vi "Pre Launch Init.vi"(11 "Vision Receiver in":refnum<class "Vision Receiver.lvclass">) -> (0 "error out":errorcluster, 3 "Vision Receiver out":refnum<class "Vision Receiver.lvclass">)   [LabVIEW 2022 SP3, in "Vision.lvlib" / "Vision Receiver.lvlib" / "Vision Receiver.lvclass"]
doc: "(<B>Filename</B>: Actor Framework.lvlib:Actor.lvclass:Pre Launch Init.vi)\n\nDefines behavior that occurs after the Launch Actor method is invoked but before the actor's Actor Core method begins running.\n\nThe Pre Launch Init method is guaranteed to finish before the Launch Actor method returns to its caller and before the actor itself receives any messages. Any references that the Pre Launch Init method obtains are guaranteed to have the same lifetime as the actor itself. Any errors that the Pre Launch Init method returns will abort the launch.\n\nBy default, this method does nothing. A descendant class may override it to define behavior."
uses:
  Vision Receiver.lvclass
  Vision Receiver.lvclass/Vision Receiver.ctl
  <vilib>/MGI/Monitored Actor/Monitored Actor/Monitored Actor/Monitored Actor.lvclass
panel:
  in  "RX Data":cluster{"RX":bool, "Data":u8[]}
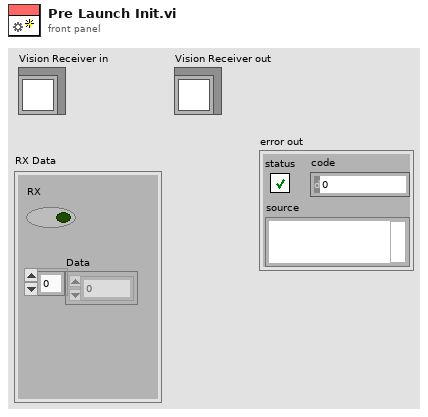
[diagram p1: front panel]
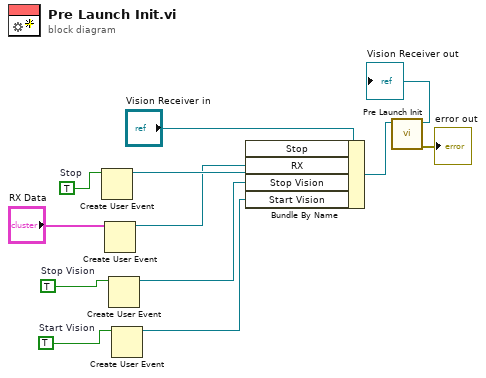
[diagram p0: block diagram]
diagram:
  w4 = TRUE  # Start Vision
  w3 = TRUE  # Stop Vision
  w10 = TRUE  # Stop
  n1 = Create User Event(user event datatype=w10) -> (user event=w9:refnum<user-event>)  [unwired: 1 in, 1 out]
  n2 = Create User Event(user event datatype="RX Data") -> (user event=w8:refnum<user-event>)  [unwired: 1 in, 1 out]
  n3 = Create User Event(user event datatype=w3) -> (user event=w2:refnum<user-event>)  [unwired: 1 in, 1 out]
  n4 = Create User Event(user event datatype=w4) -> (user event=w1:refnum<user-event>)  [unwired: 1 in, 1 out]
  n5 = Bundle By Name(cluster="Vision Receiver in", "Stop"=w9, "RX"=w8, "Stop Vision"=w2, "Start Vision"=w1) -> (w6:refnum<class "Vision Receiver.lvclass">)
  n6 = call-parent "Pre Launch Init.vi"("Monitored Actor in"=w6) -> ("error out"=→"error out":errorcluster, "Monitored Actor out"=→"Vision Receiver out":refnum<class "Vision Receiver.lvclass">)  [unwired: 9 in]
